vi "STD Cal Date Check.vi"(8 "에러 입력":errorcluster caption="에러 입력(에러 없음)") -> (0 "error out":errorcluster caption="에러 출력", 2 "비어있음?":bool, 3 "Data":string[][](array[string]))   [LabVIEW 2020]
uses:
  Controls/Cmd_Read Query.ctl
  Controls/Clst_Query Info.ctl
  <vilib>/addons/database/NI_Database_API.lvlib
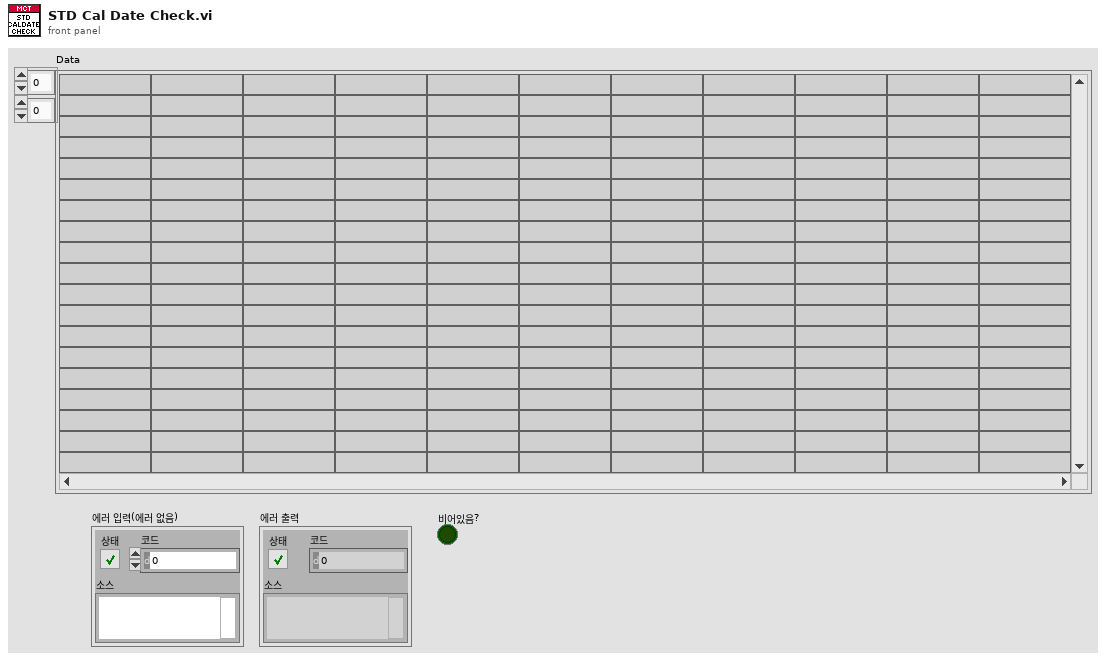
[diagram p1: front panel]
types:
  T1 = typedef "Clst_Query Info.ctl" = cluster{"사번":string, "등록번호":string, "업체명":string, "세부분류코드":string, "형식":string, "기기번호":string, "FUNC":string, "FUNC_EXT":string, "옵션":string, "추가문자열":string, "일자":string, "배열 1":string[], "배열 2":string[], "항목명":string, "문자열":string, "이름":string}
  T2 = typedef "Cmd_Read Query.ctl" = enum16{"교정자 이름 얻기", "인증교정자 얻기", "기술책임자 얻기", "기책부책 얻기", "등록번호 얻기", "등록정보 얻기", "업체정보 얻기", "교정일자(CAMAS) 얻기", "교정일자(CALSTD) 얻기", "교정환경 얻기", "교정절차서 목록 얻기", "교정절차서명 얻기", "교정절차 목록얻기", "교정절차 얻기", "PROC 교정절차 얻기", "PROC SPEC 얻기", "교정절차(Func별) 얻기", "교정절차(Func_ext별) 얻기", "기관코드 얻기", "교정기능(세부분류) 얻기", "교정기능(모델) 얻기", "교정기능 목록 얻기", "교정기능 명칭 얻기", "교정기능 항목명칭 얻기", "DB (사용기준기) 얻기", "DB (기준기이름) 얻기", "DB (기준기이름목록) 얻기", "DB (기준기목록) 얻기", "DB (기준기값) 얻기", "DB (CMC) 얻기", "DB (FUNC) 얻기", "DB (CALNAME) 얻기", "DB (STDNAME) 얻기", "DB (SPEC) 얻기", "모델(항목전체) 얻기", "모델(최대범위) 얻기", "모델(최소범위) 얻기", "모델(최대최소) 얻기", "모델(범위조건) 얻기", "모델(등록요청) 얻기", "모델(형식별) 얻기", "모델(조건별) 얻기", "모델(모델검색) 얻기", "세부분류 목록 얻기", "기준기등록리스트 얻기", "STD Cal Date Check", "DB등록일자 얻기", "적용항목 얻기", "기타정보 얻기", "기준기요청 얻기", "서버버전 얻기"}
  T3 = typedef "NI_Database_API.lvlib/Conn ObjectReference.ctl" = refnum<k1>
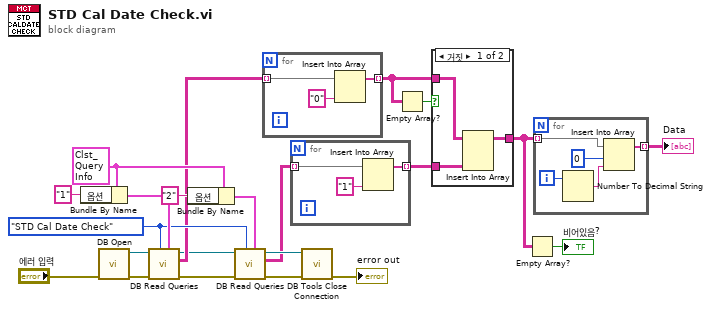
[diagram p0: block diagram]
diagram:
  w10 = T1 {"사번"="", "등록번호"="", "업체명"="", "세부분류코드"="", "형식"="", "기기번호"="", "FUNC"="", "FUNC_EXT"="", "옵션"="", "추가문자열"="", "일자"="", "배열 1"=[], "배열 2"=[], "항목명"="", "문자열"="", "이름"=""} ("Query info")
  w12 = Cmd_Read_Query."STD Cal Date Check" ("Query Command")
  n1 = Bundle By Name(cluster=w10, "옵션"="1") -> (w13:T1)
  n2 = call "DB Open.vi"("에러 입력"="에러 입력") -> ("에러 출력"=w7:errorcluster, "참조 번호 출력"=w6:T3)  [unwired: 9 in]
  n3 = call "DB Read Queries.vi"("Query info"=w13, "Query Command"=w12, "에러 입력(에러 없음)"=w7, "참조 번호 입력"=w6) -> ("에러 출력"=w5:errorcluster, "Data"=w8:string[][], "참조 번호 출력"=w2:T3)  [unwired: 3 in, 2 out]
  n4 = Bundle By Name(cluster=w10, "옵션"="2") -> (w11:T1)
  n5 = call "DB Read Queries.vi"("Query info"=w11, "Query Command"=w12, "에러 입력(에러 없음)"=w5, "참조 번호 입력"=w2) -> ("에러 출력"=w4:errorcluster, "Data"=w1:string[][], "참조 번호 출력"=w3:T3)  [unwired: 3 in, 2 out]
  n6 = for {
    tunnel: w8 -> [w25] mode=indexing
    tunnel: [w23] -> w20 mode=indexing
    n7 = Insert Into Array(array=w25, new element="0" ("새 원소/부분배열")) -> (w23:string[])  [unwired: 1 in]
  }
  n8 = for {
    tunnel: w1 -> [w28] mode=indexing
    tunnel: [w26] -> w22 mode=indexing
    n9 = Insert Into Array(array=w28, new element="1" ("새 원소/부분배열")) -> (w26:string[])  [unwired: 1 in]
  }
  n10 = call <vilib>:"DB Tools Close Connection.vi"("error in (no error)"=w4, "connection reference"=w3) -> ("error out"=→"error out":errorcluster)  [unwired: 5 in]
  n11 = Empty Array?(array=w20) -> (empty?=w21:bool)
  n12 = case shown="거짓" w21 {
    tunnel: w22 -> [w31 w32]
    tunnel: w20 -> [w30 _]
    tunnel: [w29 w32] -> w16
    frame False {
      n13 = Insert Into Array(array=w30, new element=w31) -> (w29:string[][])  [unwired: 2 in]
    }
    frame True {
    }
  }
  n14 = Empty Array?(array=w16) -> (empty?=→"비어있음?":bool)
  n15 = for {
    tunnel: w16 -> [w37] mode=indexing
    tunnel: [w33] -> w15 mode=indexing
    i -> [w36]
    n16 = Number To Decimal String(number=w36) -> (decimal integer string=w35:string)  [unwired: 1 in]
    n17 = Insert Into Array(array=w37, index=0 ("인덱스"), new element=w35) -> (w33:string[])
  }
  "Data" <- w15
